vi "6_1_2_3_ARRAYS.vi"() -> ()   [LabVIEW 2026]
uses:
  <vilib>/Analysis/Matrix/Datatypes/RealMatrix.ctl
  <vilib>/numeric/Random Number (Range) I64.vi
  <vilib>/numeric/Random Number (Range) DBL.vi
  <vilib>/numeric/sub_Random U32.vi
  <vilib>/Analysis/Matrix/Numeric/Conversions/Array To Matrix - RA.vi
  <vilib>/Analysis/Matrix/Numeric/Multiply/Multiply - RM,RM.vi
  <vilib>/Analysis/Matrix/NI_Matrix.lvlib
panel:
  out "DESC SORTED":dbl[](array[numeric])
  out "ASC SORTED":dbl[](array[numeric])
  out "1D-ARRAY":dbl[](array[numeric])
  out "A*B":dbl[][](array[numeric])
  in  "B":dbl[][](array[numeric])
  in  "A":dbl[][](array[numeric])
  out "A * B":T1
  out "Array 3":dbl[](array[numeric])
  out "Array 2":dbl[](array[numeric])
  out "Array":dbl[](array[numeric])
  in  "Numeric 2":dbl
  in  "Numeric":dbl
  # "3x3 matrix multiplication"
  # "arrange nums in asc and desc order"
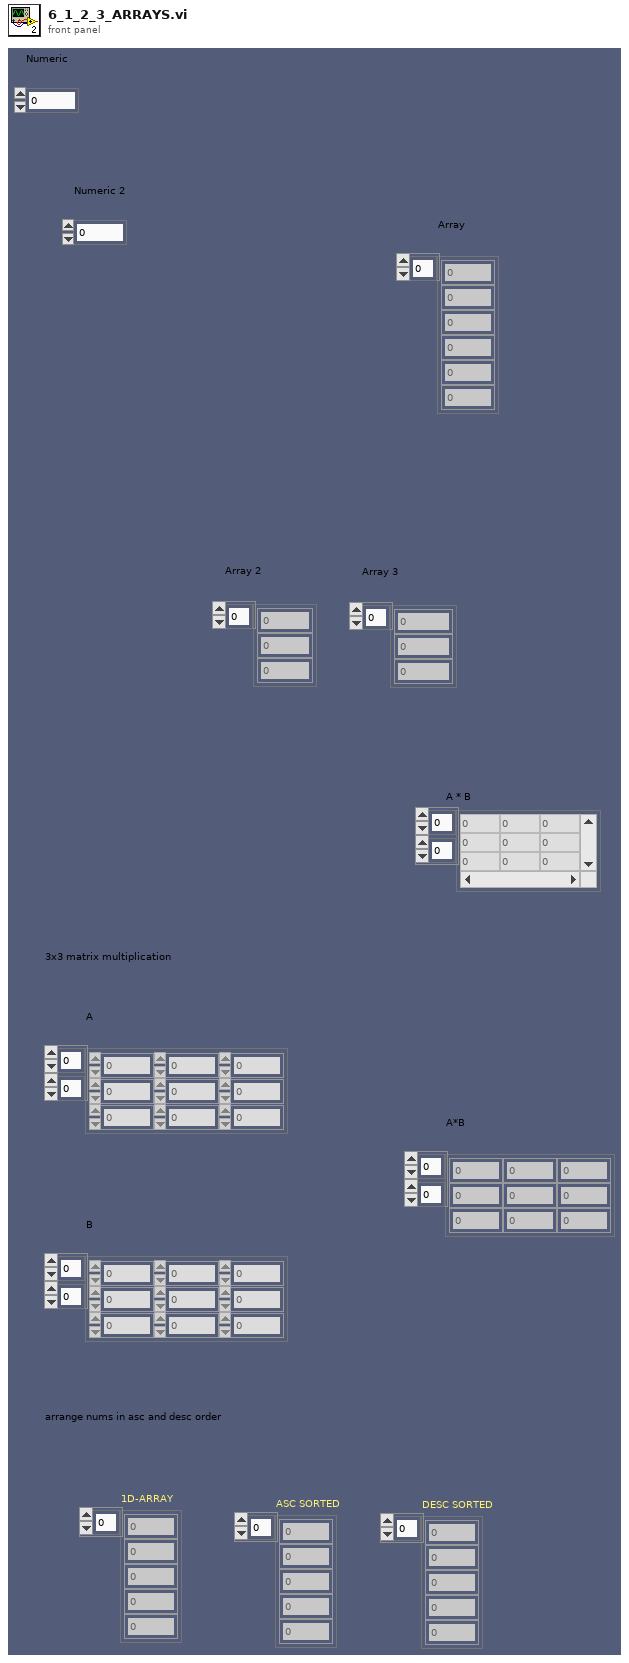
[diagram p1: front panel]
types:
  T1 = typedef "NI_Matrix.lvlib/RealMatrix.ctl" = dbl[][]
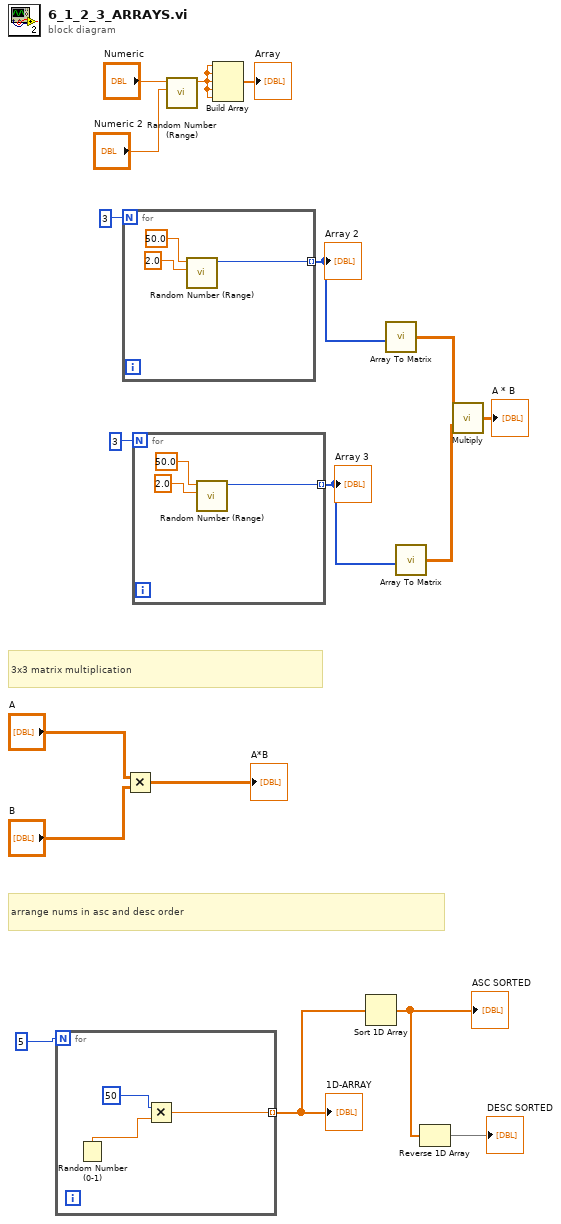
[diagram p0: block diagram]
diagram:
  # "3x3 matrix multiplication"
  # "arrange nums in asc and desc order"
  n1 = for {
    N: 5 -> [_]
    tunnel: [w19] -> w3 mode=indexing
    n2 = Random Number (0-1)() -> (number: 0 to 1=w21:dbl)
    n3 = Multiply(x=50, y=w21) -> (x*y=w19:dbl)
  }
  "1D-ARRAY" <- w3
  n4 = for {
    N: 3 -> [_]
    tunnel: [w22] -> w13 mode=indexing
    n5 = call-poly <vilib>:"Random Number (Range).vi"("lower bound (-100)"=2.0 ("lower bound (0)"), "upper bound (100)"=50.0) -> ("number"=w22:i64)  [unwired: 9 in]
  }
  "Array 2" <- w13
  n6 = Multiply(x="A", y="B") -> (x*y=→"A*B":dbl[][])
  n7 = for {
    N: 3 -> [_]
    tunnel: [w25] -> w11 mode=indexing
    n8 = call-poly <vilib>:"Random Number (Range).vi"("lower bound (-100)"=2.0 ("lower bound (0)"), "upper bound (100)"=50.0) -> ("number"=w25:i64)  [unwired: 9 in]
  }
  "Array 3" <- w11
  n9 = call-poly <vilib>:"Random Number (Range).vi"("lower bound (0)"="Numeric 2", "upper bound (100)"="Numeric") -> ("number"=w15:dbl)  [unwired: 9 in]
  n10 = Build Array(w15, w15, w15, w15, w15) -> (→"Array":dbl[])
  n11 = Sort 1D Array(array=w3) -> (sorted array=w2:dbl[])
  "ASC SORTED" <- w2
  n12 = call-poly <vilib>:"Array To Matrix.vi"("Real 1D Array"=w13) -> ("Real Matrix (Column Vector)"=w10:T1)
  n13 = call-poly <vilib>:"Array To Matrix.vi"("Real 1D Array"=w11) -> ("Real Matrix (Column Vector)"=w9:T1)
  n14 = Reverse 1D Array(array=w2) -> (reversed array=→"DESC SORTED":dbl[])
  n15 = call-poly <vilib>:"Multiply.vi"("Real Matrix B"=w9, "Real Matrix A"=w10) -> ("A * B"=→"A * B":T1)
